vi "Set Exclusions.vi"(8 "error in (no error)":errorcluster, 10 "Exclusions":refnum<vi>[](array[refnum]), 11 "Dialog in":refnum<class "Dialog.lvclass">) -> (0 "error out":errorcluster, 3 "Dialog out":refnum<class "Dialog.lvclass">)   [LabVIEW 2012, in "Dialog.lvlib" / "Dialog.lvclass"]
uses:
  Dialog.lvclass
  Dialog.lvclass/Dialog.ctl
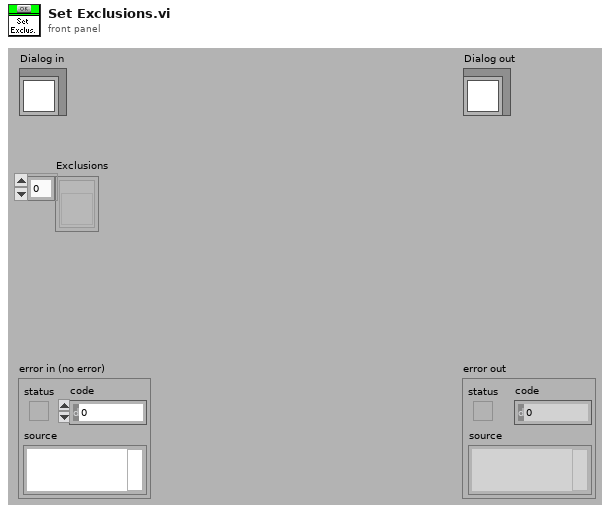
[diagram p1: front panel]
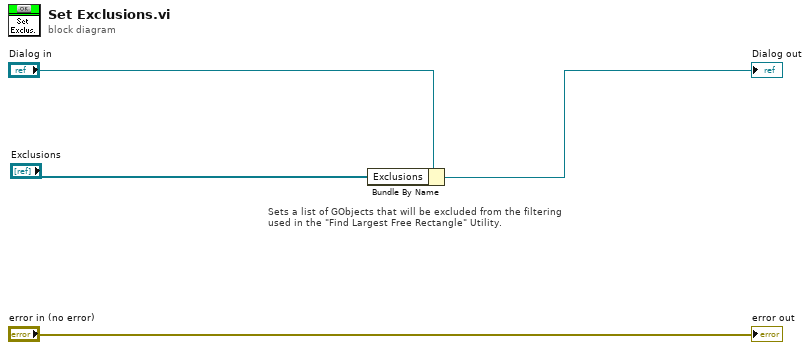
[diagram p0: block diagram]
diagram:
  # "Sets a list of GObjects that will be excluded from the filtering\nused in the \"Find Largest Free Rectangle\" Utility."
  n1 = Bundle By Name(cluster="Dialog in", "Exclusions"="Exclusions") -> (→"Dialog out":refnum<class "Dialog.lvclass">)
  "error out" <- "error in (no error)"
